vi "SVT STFT vs Time (Colormap).vi"(0 "scaled signal [EU]":waveform(dbl), 5 "FFT block size":i32=1024 min=1, 7 "window":T9(ring)=enum."Hanning", 9 "time segment":T8={"from [s]"=-1.0, "to [s]"=-1.0, "time increment"=100.0, "time increment units (%)"=enum."%"} {"time increment" format="%.2f"; "to [s]" format="%.2f"; "from [s]" format="%.2f"}, 11 "error in (no error)":errorcluster, 12 "dB On (T)":bool=TRUE, 13 "weighting":u16(ring) items=["Linear", "A-weighting", "B-weighting", "C-weighting"]) -> (4 "colormap":T7, 6 "unit label":string, 14 "spectrum info":T1={"channel name"="", "description"="", "x-axis units"=0, "spectral info"={"spectrum type"=enum."Power [Magnitude^2]", "linear/dB"=enum."linear", "window"=0, "window size"=0, "FFT size"=0}, "engineering units"=0, "custom label"="", "dB reference [EU]"=0.0, "peak units"=enum."rms", "weighting filter"=0, "spectral density?"=FALSE, "unit label"="", "spectrum skewed?"=FALSE, "complimentary spectrum units"=enum."none"} {"x-axis units" items=["Time (s)"=0, "Frequency-CB (Hz)"=1, "Frequency-CPB (Hz)"=1248, "Frequency-Arbitrary (Hz)"=2357, "Quefrency (s)"=2, "Revolutions (rev)"=3, "Order"=4, "Speed (RPM)"=11, "Speed (rad/s)"=21, "Index"=65535]; "weighting filter" items=["Linear", "A-weighting", "B-weighting", "C-weighting", "ITU-R 468-4", "Dolby", "CCITT", "C-message", "Wb", "Wc", "Wd", "We", "Wf", "Wh", "Wj", "Wk", "Wm", "AES17 20 kHz lowpass", "AES17 40 kHz lowpass", "AES17 20 kHz highpass", "AES17 40 kHz highpass"]; "dB reference [EU]" format="%.2f"; "engineering units" items=["custom..."=0, "V"=1, "A"=21, "C"=30, "pC"=31, "s"=32, "-"=29, "Pa"=2, "N"=20, "g"=3, "m/s^2"=4, "m/s"=5, "m"=6, "mm/s"=12, "mm"=13, "micron/s"=14, "micron"=15, "in/s^2"=7, "in/s"=8, "in"=9, "mil/s"=10, "mil"=11, "rad/s^2"=16, "rad/s"=17, "rad"=18, "deg/s^2"=26, "deg/s"=27, "deg"=28, "RPM"=22, "cycle/s^2"=23, "Hz"=24, "cycle"=25, "strain"=19]; "spectral info"."window" items=["None "=0, "Hanning"=1, "Hamming"=2, "Blackman-Harris"=3, "Exact Blackman"=4, "Blackman"=5, "Flat Top"=6, "4 Term B-Harris "=7, "7 Term B-Harris"=8, "Low Sidelobe"=9, "Force - Exponential"=10, "Gaussian"=62]}, 15 "error out":errorcluster)   [LabVIEW 2017, in "SoundVib_Transient.lvlib"]
doc: "Performs a short-time Fourier transform (STFT) on <B>scaled signal [EU]</B> and returns the power spectrum, waterfall, or colormap at the various times you specify. Wire data to the <B>scaled signal [EU]</B> input to determine the polymorphic instance to use or manually select the instance."
uses:
  <vilib>/addons/Sound and Vibration/svt_Transients/SoundVib_Transient.lvlib
  <vilib>/addons/_NISVFA/_Shared subVIs/Controls/svc_Spectrum Info.ctl
  <vilib>/addons/_NISVFA/_Shared subVIs/Controls/svc_X-Axis Units.ctl
  <vilib>/addons/_NISVFA/_Shared subVIs/Controls/svc_Spectrum Type.ctl
  <vilib>/addons/_NISVFA/_Shared subVIs/Controls/svc_Engineering Units Text Ring.ctl
  <vilib>/addons/_NISVFA/_Shared subVIs/Controls/svc_Weighting Filter Text Ring.ctl
  <vilib>/addons/_NISVFA/_Shared subVIs/Controls/svc_Complimentary Spectrum Units.ctl
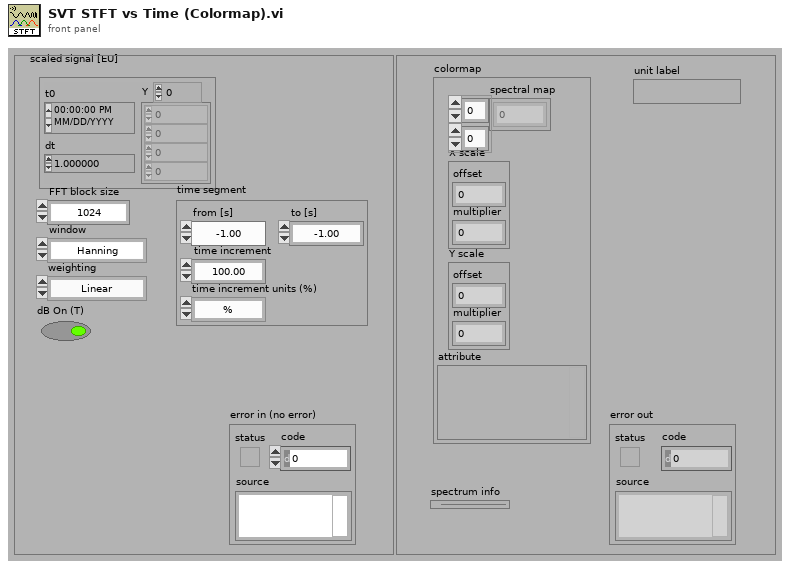
[diagram p1: front panel]
types:
  T1 = typedef "svc_Spectrum Info.ctl" = cluster{"channel name":string, "description":string, "x-axis units":T2, "spectral info":cluster{"spectrum type":T3, "linear/dB":enum16{"linear", "dB"}, "window":u16, "window size":i32, "FFT size":i32}, "engineering units":T4, "custom label":string, "dB reference [EU]":dbl, "peak units":enum16{"rms", "peak", "peak-peak"}, "weighting filter":T5, "spectral density?":bool, "unit label":string, "spectrum skewed?":bool, "complimentary spectrum units":T6}
  T2 = typedef "svc_X-Axis Units.ctl" = u16
  T3 = typedef "svc_Spectrum Type.ctl" = enum16{"FFT Spectrum [complex]", "Amplitude [Magnitude]", "Power [Magnitude^2]", "Cross Spectrum [complex]", "Frequency Response [Complex]"}
  T4 = typedef "svc_Engineering Units Text Ring.ctl" = u16
  T5 = typedef "svc_Weighting Filter Text Ring.ctl" = u16
  T6 = typedef "svc_Complimentary Spectrum Units.ctl" = enum16{"none", "radians", "degrees", "cycles", "imaginary"}
  T7 = cluster{"spectral map":dbl[][], "X scale":cluster{"offset":dbl, "multiplier":dbl}, "Y scale":cluster{"offset":dbl, "multiplier":dbl}, "attribute":variant}
  T8 = cluster{"from [s]":dbl, "to [s]":dbl, "time increment":dbl, "time increment units (%)":enum16{"%", "s", "ms"}}
  T9 = enum16{"None ", "Hanning", "Hamming", "Blackman-Harris", "Exact Blackman", "Blackman", "Flat Top", "4 Term B-Harris ", "7 Term B-Harris", "Low Sidelobe"}
  T10 = enum16{"Frequency-Time", "Time-Frequency", "Order-Time", "Time-Order", "Frequency-RPM", "RPM-Frequency", "Order-RPM", "RPM-Order"}
  T11 = cluster{"FFT block size":i32, "number of FFT":i32, "start index":i32, "increment":dbl}
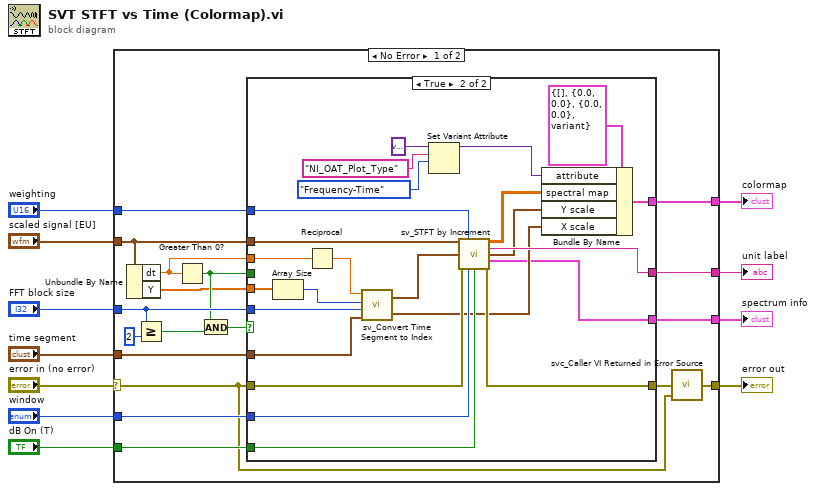
[diagram p0: block diagram]
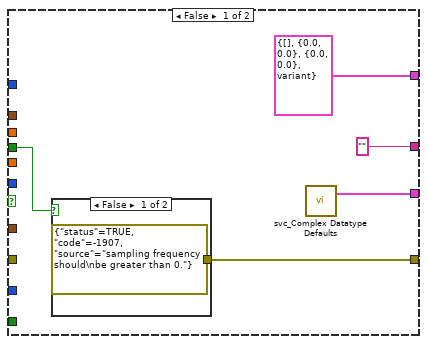
[diagram p2: hidden frame]
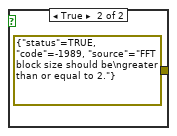
[diagram p3: hidden frame]
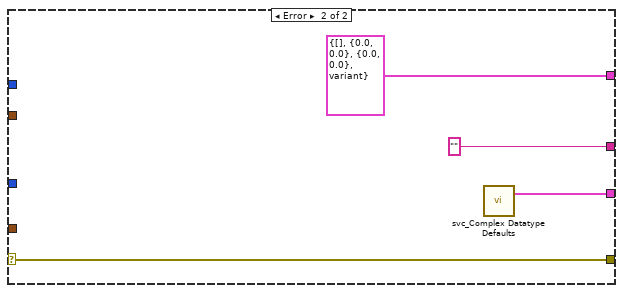
[diagram p4: hidden frame]
diagram:
  n1 = case shown="No Error" "error in (no error)" {
    selector: "error in (no error)" -> [w14 w64]
    tunnel: "dB On (T)" -> [w27 _]
    tunnel: "window" -> [w28 _]
    tunnel: "FFT block size" -> [w24 _]
    tunnel: "time segment" -> [w29 _]
    tunnel: "scaled signal [EU]" -> [w20 _]
    tunnel: [w21 w64] -> w5
    tunnel: [w25 "" ("unit label")] -> w4
    tunnel: "weighting" -> [w26 _]
    tunnel: [w13 T7 {"spectral map"=[], "X scale"={"offset"=0.0, "multiplier"=0.0}, "Y scale"={"offset"=0.0, "multiplier"=0.0}, "attribute"=variant} ("Colormap 2")] -> w2
    tunnel: [w12 w61] -> w1
    frame No Error {
      n2 = Unbundle By Name(w20) -> ("dt"=w16:dbl, "Y"=w15:dbl[])
      n3 = Greater Or Equal?(x=w24, y=2) -> (x >= y?=w19:bool)
      n4 = Greater Than 0?(x=w16) -> (x > 0?=w17:bool)
      n5 = And(x=w17, y=w19) -> (x .and. y?=w18:bool)
      n6 = case shown="True" w18 {
        tunnel: w24 -> [_ w59]
        tunnel: w29 -> [_ w58]
        tunnel: w28 -> [_ w56]
        tunnel: w27 -> [_ w55]
        tunnel: w26 -> [_ w54]
        tunnel: ["" ("unit label") w53] -> w25
        tunnel: w20 -> [_ w52]
        tunnel: w14 -> [_ w50]
        tunnel: [w34 w49] -> w22
        tunnel: w17 -> [w32 _]
        tunnel: w16 -> [_ w48]
        tunnel: w15 -> [_ w47]
        tunnel: [T7 {"spectral map"=[], "X scale"={"offset"=0.0, "multiplier"=0.0}, "Y scale"={"offset"=0.0, "multiplier"=0.0}, "attribute"=variant} ("Colormap 2") w45] -> w13
        tunnel: [w30 w37] -> w12
        frame False {
          n7 = case shown="False" w32 {
            tunnel: [errorcluster {"status"=TRUE, "code"=-1907, "source"="sampling frequency should\nbe greater than 0."} ("error out") errorcluster {"status"=TRUE, "code"=-1989, "source"="FFT block size should be\ngreater than or equal to 2."} ("error out")] -> w34
            frame False {
            }
            frame True {
            }
          }
          n8 = call <vilib>:"svc_Complex Datatype Defaults.vi"() -> ("dead spectrum info"=w30:T1)  [unwired: 11 in, 8 out]
        }
        frame True {
          n9 = Array Size(array=w47) -> (size(s)=w60:i32)
          n10 = Reciprocal(x=w48) -> (1/x=w51:dbl)
          n11 = call <vilib>:"sv_Convert Time Segment to Index.vi"("sampling frequency [Hz]"=w51, "array size"=w60, "FFT block size"=w59, "time segment"=w58) -> ("FFT info"=w57:T11, "to and delta t [s]"=w39:cluster{"to":dbl, "delta t":dbl})  [unwired: 1 in]
          n12 = Set Variant Attribute(Variant=variant ("variant"), name="NI_OAT_Plot_Type", value=T10."Frequency-Time" ("plot type")) -> (Variant out=w41:variant)  [unwired: 1 in, 2 out]
          n13 = call <vilib>:"sv_STFT by Increment.vi"("scaled signal [EU]"=w52, "weighting filter"=w54, "FFT info"=w57, "error in (no error)"=w50, "window"=w56, "dB On (T)"=w55) -> ("power spectra [dB EU]"=w40:dbl[][], "unit label"=w53:string, "f0 and delta f [Hz]"=w38:cluster{"f0":dbl, "delta f":dbl}, "spectrum info"=w37:T1, "error out"=w49:errorcluster)  [unwired: 5 in]
          n14 = Bundle By Name(cluster=T7 {"spectral map"=[], "X scale"={"offset"=0.0, "multiplier"=0.0}, "Y scale"={"offset"=0.0, "multiplier"=0.0}, "attribute"=variant} ("Colormap 2"), "attribute"=w41, "spectral map"=w40, "Y scale"=w38, "X scale"=w39) -> (w45:T7)
        }
      }
      n15 = call <vilib>:"svc_Caller VI Returned in Error Source.vi"("warning input to caller"=w14, "error in (no error)"=w22) -> ("error out"=w21:errorcluster)  [unwired: 3 in]
    }
    frame Error {
      n16 = call <vilib>:"svc_Complex Datatype Defaults.vi"() -> ("dead spectrum info"=w61:T1)  [unwired: 11 in, 8 out]
    }
  }
  "error out" <- w5
  "unit label" <- w4
  "colormap" <- w2
  "spectrum info" <- w1
